vi "TWritePIStageSettings.vi"(1 "error in (no error)":errorcluster) -> (0 "error out":errorcluster)   [LabVIEW 2009]
uses:
  StageSettings.ctt
  <vilib>/Utility/config.llb/NI_LVConfig.lvlib
panel:
  out "PI Stage Setup":T1={"channels (x, y, z)"="2", "Stage Scaling (V/µm)"=0.1} {"Stage Scaling (V/µm)" format="%.2f"}
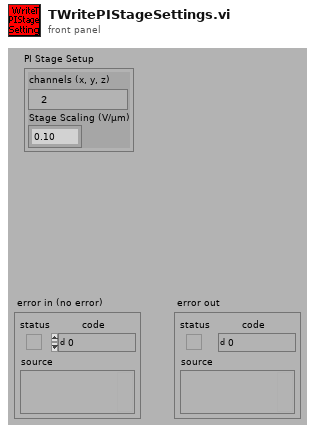
[diagram p1: front panel]
types:
  T1 = typedef "StageSettings.ctt" = cluster{"channels (x, y, z)":tag, "Stage Scaling (V/µm)":dbl}
  T2 = typedef "NI_LVConfig.lvlib/Config Data RefNum.ctl" = refnum<k1>
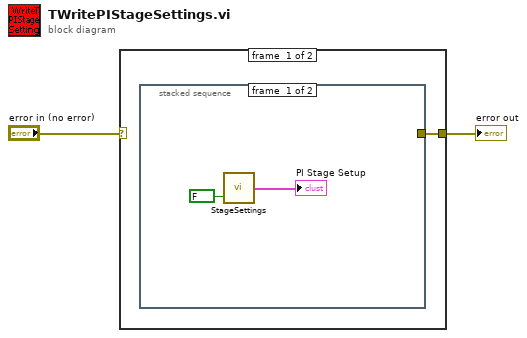
[diagram p0: block diagram]
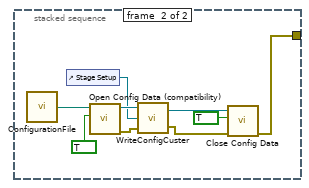
[diagram p2: hidden frame]
diagram:
  n1 = case shown="No Error" "error in (no error)" {
    selector: "error in (no error)" -> [_ w15]
    tunnel: [w3 w15] -> w1
    frame #0 {
      n2 = stacked-sequence {
        tunnel: [_ w6] -> w3
        frame #0 {
          n3 = call "StageSettings.vi"("Get/Set"=FALSE) -> ("PI Stage Setup (output)"=→"PI Stage Setup":T1)  [unwired: 1 in]
        }
        frame #1 {
          n4 = call "ConfigurationFile.vi"() -> ("Configuration File (output)"=w10:path)  [unwired: 2 in]
          n5 = control-ref of="Stage Setup"() -> (w9:refnum<vi>)
          n6 = call <vilib>:"Open Config Data (compatibility).vi"("create file if necessary (T)"=TRUE ("create file if necessary? (T)"), "configuration file path"=w10) -> ("error out"=w12:errorcluster, "refnum"=w13:T2)  [unwired: 7 in, 1 out]
          n7 = call "WriteConfigCuster.vi"("error in (no error)"=w12, "Ctrl Reference"=w9, "ConfigFile (input)"=w13) -> ("error out"=w7:errorcluster, "ConfigFile (output)"=w8:T2)
          n8 = call "Close Config Data.vi"("error in (no error)"=w7, "write configuration file? (T)"=TRUE ("write configuration file? (F)"), "refnum"=w8) -> ("error out"=w6:errorcluster)  [unwired: 8 in]
        }
      }
    }
    frame #1 {
    }
  }
  "error out" <- w1
